vi "Cargo Manip Control.vi"() -> ()   [LabVIEW 2018]
uses:
  <vilib>/Rock Robotics/WPI/DriverStation/WPI_DriverStationDerivedRobotMode.ctl
  SubSystems/Controllers/Manipulator Controlller/Manipulator Controller Global.vi
  SubSystems/Cargo Intake/Cargo Intake Global.vi
  SubSystems/Lift/Lift Global.vi
panel:
  out "Fun Thing":bool
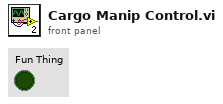
[diagram p1: front panel]
types:
  T1 = typedef "WPI_DriverStationDerivedRobotMode.ctl" = enum16{"Init", "Execute", "Stop"}
  T2 = enum16{"Hatch Panel Zone 1", "Hatch Panel Zone 2", "Hatch Panel Zone 3", "Cargo Zone 1", "Cargo Zone 2", "Cargo Zone 3", "Cargo Ship Zone"}
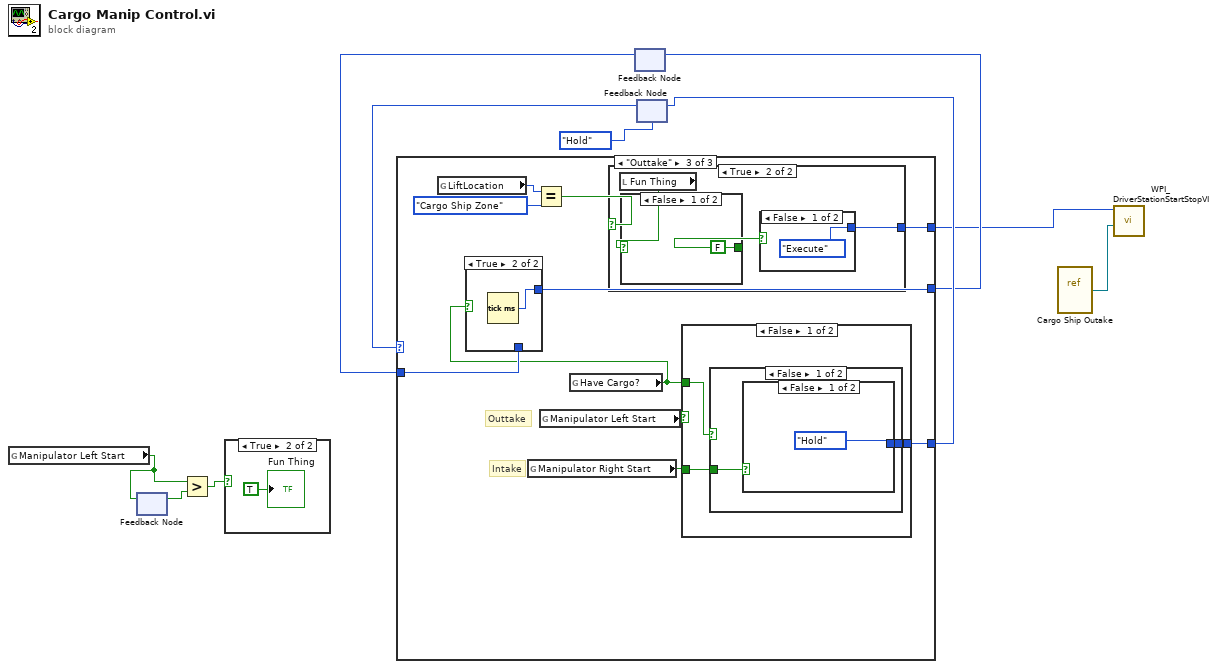
[diagram p0: block diagram]
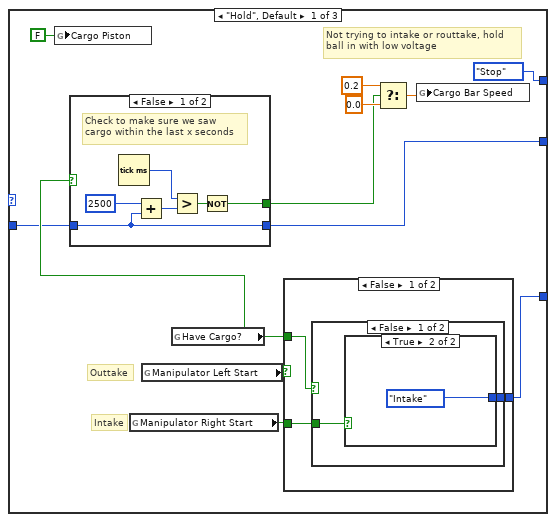
[diagram p3: hidden frame]
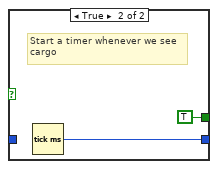
[diagram p4: hidden frame]
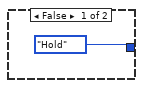
[diagram p5: hidden frame]
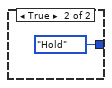
[diagram p6: hidden frame]
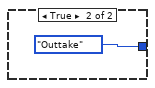
[diagram p7: hidden frame]
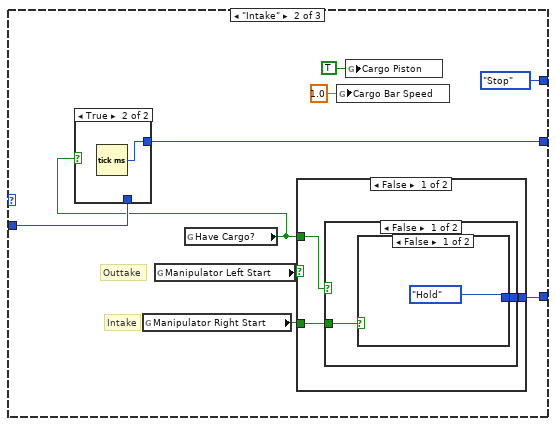
[diagram p8: hidden frame]
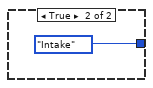
[diagram p10: hidden frame]
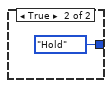
[diagram p11: hidden frame]
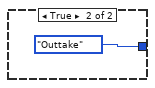
[diagram p12: hidden frame]
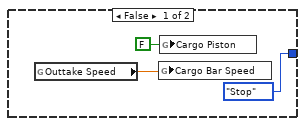
[diagram p13: hidden frame]
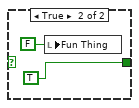
[diagram p14: hidden frame]
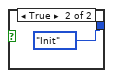
[diagram p15: hidden frame]
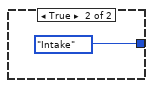
[diagram p17: hidden frame]
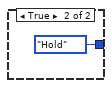
[diagram p18: hidden frame]
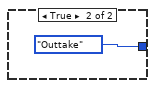
[diagram p19: hidden frame]
diagram:
  n1 = global read "Manipulator Controller Global.vi" "Manipulator Left Start"() -> (w2:bool)
  n2 = feedback #1() -> (w3:bool)  [unwired: 1 in]
  n3 = feedback-in #1(w2) -> ()
  n4 = Greater?(x=w2, y=w3) -> (0:w1:bool)
  n5 = case shown="True" w1 {
    frame False {
    }
    frame True {
      "Fun Thing" <- TRUE ("Fun Thing")
    }
  }
  n6 = feedback #2() -> (w6:u32)  [unwired: 1 in]
  n7 = feedback #3(enum16{"Going Up", "Outtake", "Intake", "Hold"}."Hold") -> (w9:enum16{"Going Up", "Outtake", "Intake", "Hold"})
  n8 = case shown="\"Outtake\"" w9 {
    tunnel: [w21 w45 w68] -> w8
    tunnel: [w16 w43 w66] -> w7
    tunnel: w6 -> [w14 w44 w67]
    tunnel: [WPI_DriverStationDerivedRobotMode."Stop" ("Call Context") WPI_DriverStationDerivedRobotMode."Stop" ("Call Context") w61] -> w4
    frame "Hold", Default {
      # "Outtake"
      # "Intake"
      # "Not trying to intake or routtake, hold\nball in with low voltage"
      n9 = global write "Cargo Intake Global.vi" "Cargo Piston"(FALSE ("Cargo Piston")) -> ()
      n10 = global read "Manipulator Controller Global.vi" "Manipulator Right Start"() -> (w23:bool)
      n11 = global read "Manipulator Controller Global.vi" "Manipulator Left Start"() -> (w22:bool)
      n12 = global read "Cargo Intake Global.vi" "Have Cargo?"() -> (w15:bool)
      n13 = case shown="False" w15 {
        tunnel: [w29 w31] -> w16
        tunnel: w14 -> [w29 _]
        tunnel: [w24 TRUE] -> w13
        frame False {
          # "Check to make sure we saw \ncargo within the last x seconds"
          n14 = Tick Count (ms)() -> (millisecond timer value=w26:u32)
          n15 = Add(x=u32 2500, y=w29) -> (x+y=w27:u32)
          n16 = Greater?(x=w26, y=w27) -> (0:w25:bool)
          n17 = Not(x=w25) -> (.not. x?=w24:bool)
        }
        frame True {
          # "Start a timer whenever we see\ncargo"
          n18 = Tick Count (ms)() -> (millisecond timer value=w31:u32)
        }
      }
      n19 = case shown="False" w22 {
        tunnel: w23 -> [w34 _]
        tunnel: [w33 enum16{"Going Up", "Outtake", "Intake", "Hold"}."Outtake"] -> w21
        tunnel: w15 -> [w32 _]
        frame False {
          n20 = case shown="False" w32 {
            tunnel: w34 -> [w36 _]
            tunnel: [w35 enum16{"Going Up", "Outtake", "Intake", "Hold"}."Hold"] -> w33
            frame False {
              n21 = case shown="True" w36 {
                tunnel: [enum16{"Going Up", "Outtake", "Intake", "Hold"}."Hold" enum16{"Going Up", "Outtake", "Intake", "Hold"}."Intake"] -> w35
                frame False {
                }
                frame True {
                }
              }
            }
            frame True {
            }
          }
        }
        frame True {
        }
      }
      n22 = Select(t=0.2, s=w13, f=0.0) -> (s? t:f=w19:dbl)
      n23 = global write "Cargo Intake Global.vi" "Cargo Bar Speed"(w19) -> ()
    }
    frame "Intake" {
      # "Outtake"
      # "Intake"
      n24 = global read "Manipulator Controller Global.vi" "Manipulator Right Start"() -> (w49:bool)
      n25 = global read "Manipulator Controller Global.vi" "Manipulator Left Start"() -> (w48:bool)
      n26 = global read "Cargo Intake Global.vi" "Have Cargo?"() -> (w42:bool)
      n27 = case shown="True" w42 {
        tunnel: w44 -> [w50 _]
        tunnel: [w50 w51] -> w43
        frame False {
        }
        frame True {
          n28 = Tick Count (ms)() -> (millisecond timer value=w51:u32)
        }
      }
      n29 = case shown="False" w48 {
        tunnel: w49 -> [w54 _]
        tunnel: [w53 enum16{"Going Up", "Outtake", "Intake", "Hold"}."Outtake"] -> w45
        tunnel: w42 -> [w52 _]
        frame False {
          n30 = case shown="False" w52 {
            tunnel: w54 -> [w56 _]
            tunnel: [w55 enum16{"Going Up", "Outtake", "Intake", "Hold"}."Hold"] -> w53
            frame False {
              n31 = case shown="False" w56 {
                tunnel: [enum16{"Going Up", "Outtake", "Intake", "Hold"}."Hold" enum16{"Going Up", "Outtake", "Intake", "Hold"}."Intake"] -> w55
                frame False {
                }
                frame True {
                }
              }
            }
            frame True {
            }
          }
        }
        frame True {
        }
      }
      n32 = global write "Cargo Intake Global.vi" "Cargo Bar Speed"(1.0 ("Cargo Bar Speed")) -> ()
      n33 = global write "Cargo Intake Global.vi" "Cargo Piston"(TRUE ("Cargo Piston")) -> ()
    }
    frame "Outtake" {
      # "Outtake"
      # "Intake"
      n34 = global read "Lift Global.vi" "LiftLocation"() -> (w64:T2)
      n35 = global read "Manipulator Controller Global.vi" "Manipulator Right Start"() -> (w70:bool)
      n36 = Equal?(x=w64, y=T2."Cargo Ship Zone") -> (x = y?=w62:bool)
      n37 = global read "Manipulator Controller Global.vi" "Manipulator Left Start"() -> (w69:bool)
      n38 = global read "Cargo Intake Global.vi" "Have Cargo?"() -> (w65:bool)
      n39 = case shown="True" w65 {
        tunnel: w67 -> [w82 _]
        tunnel: [w82 w83] -> w66
        frame False {
        }
        frame True {
          n40 = Tick Count (ms)() -> (millisecond timer value=w83:u32)
        }
      }
      n41 = case shown="True" w62 {
        tunnel: [WPI_DriverStationDerivedRobotMode."Stop" ("Call Context") w76] -> w61
        frame False {
          n42 = global read "Cargo Intake Global.vi" "Outtake Speed"() -> (w72:dbl)
          n43 = global write "Cargo Intake Global.vi" "Cargo Bar Speed"(w72) -> ()
          n44 = global write "Cargo Intake Global.vi" "Cargo Piston"(FALSE ("Cargo Piston")) -> ()
        }
        frame True {
          n45 = local read "Fun Thing"() -> (w75:bool)
          n46 = case shown="False" w75 {
            tunnel: [FALSE TRUE] -> w74
            frame False {
            }
            frame True {
              n47 = local write "Fun Thing"(FALSE ("Fun Thing")) -> ()
            }
          }
          n48 = case shown="False" w74 {
            tunnel: [WPI_DriverStationDerivedRobotMode."Execute" ("Call Context") WPI_DriverStationDerivedRobotMode."Init" ("Call Context")] -> w76
            frame False {
            }
            frame True {
            }
          }
        }
      }
      n49 = case shown="False" w69 {
        tunnel: w70 -> [w86 _]
        tunnel: [w85 enum16{"Going Up", "Outtake", "Intake", "Hold"}."Outtake"] -> w68
        tunnel: w65 -> [w84 _]
        frame False {
          n50 = case shown="False" w84 {
            tunnel: w86 -> [w88 _]
            tunnel: [w87 enum16{"Going Up", "Outtake", "Intake", "Hold"}."Hold"] -> w85
            frame False {
              n51 = case shown="False" w88 {
                tunnel: [enum16{"Going Up", "Outtake", "Intake", "Hold"}."Hold" enum16{"Going Up", "Outtake", "Intake", "Hold"}."Intake"] -> w87
                frame False {
                }
                frame True {
                }
              }
            }
            frame True {
            }
          }
        }
        frame True {
        }
      }
    }
  }
  n52 = feedback-in #2(w7) -> ()
  n53 = feedback-in #3(w8) -> ()
  n54 = vi-ref "Cargo Ship Outake.vi"() -> (w5:refnum<vi>)
  n55 = call <vilib>:"WPI_DriverStationStartStopVI.vi"("VI in"=w5, "Call Context"=w4) -> ()  [unwired: 10 in]
